vi "Get Last Error.vi"(8 "error in (no error)":errorcluster, 10 "Session Name in":string, 11 "Data Logging Manager Ref in":T1) -> (0 "error out":errorcluster, 1 "Last Error":errorcluster, 2 "Session Name out":string, 3 "Data Logging Manager Ref out":T1)   [LabVIEW 2020, in "NI_VS Data Logging API.lvlib"]
doc: "Gets the last error returned by the data logging specification specified by <B>Session Name in</B>."
uses:
  <vilib>/NI VeriStand/Execution/DataLogging/NI_VS Data Logging API.lvlib
  <vilib>/NI VeriStand/Execution/DataLogging/IDataLogging Ref.ctl
  NationalInstruments.VeriStand.ClientAPI
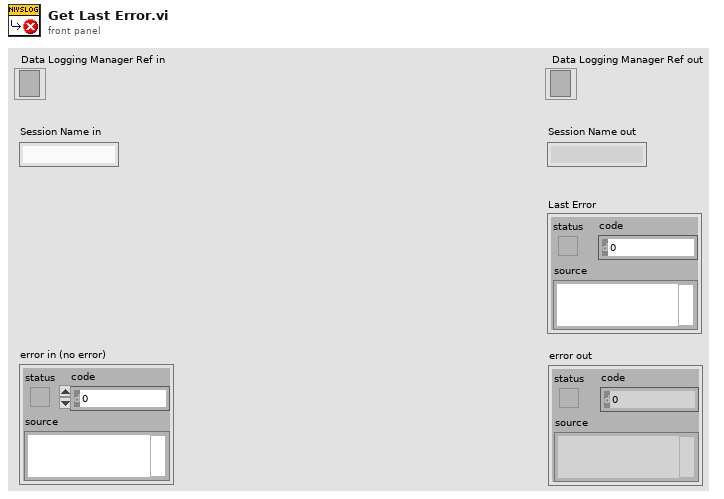
[diagram p1: front panel]
types:
  T1 = typedef "NI_VS Data Logging API.lvlib/IDataLogging Ref.ctl" = refnum<k24>
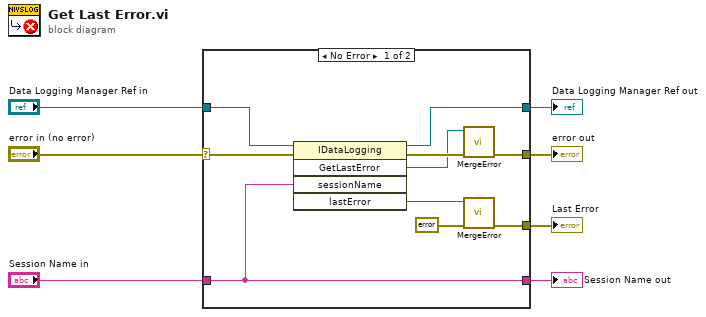
[diagram p0: block diagram]
diagram:
  n1 = case shown="No Error" "error in (no error)" {
    selector: "error in (no error)" -> [w15 w20]
    tunnel: [w12 w20] -> w6
    tunnel: [w11 w19] -> w5
    tunnel: "Data Logging Manager Ref in" -> [w17 w19]
    tunnel: [w16 w18] -> w3
    tunnel: "Session Name in" -> [w16 w18]
    tunnel: [w9 _] -> w1
    frame No Error {
      n2 = invoke class="IDataLogging" method="GetLastError"(reference=w17, error in=w15, "sessionName"=w16) -> (reference out=w11:T1, error out=w14:errorcluster, "GetLastError"=w13:refnum<k24>, "lastError"=w10:refnum<k24>)  [unwired: 2 in, 1 out]
      n3 = call <vilib>:"MergeError.vi"("error in (no error)"=w14, "Error"=w13) -> ("error out"=w12:errorcluster)  [unwired: 9 out]
      n4 = call <vilib>:"MergeError.vi"("error in (no error)"=errorcluster {"status"=FALSE, "code"=0, "source"=""}, "Error"=w10) -> ("error out"=w9:errorcluster)  [unwired: 9 out]
    }
    frame Error {
    }
  }
  "Data Logging Manager Ref out" <- w5
  "error out" <- w6
  "Session Name out" <- w3
  "Last Error" <- w1
